vi "g2.vi"() -> ()   [LabVIEW 2020]
uses:
  <vilib>/Math Plots/2D Math Plots/2D Error Bar/2D Error Bar XCtrl/2D Error Bar.xctl
  C:/Program Files/Dotfast Consulting/Timetag Explorer 2.26/ttInterface.dll
  Program Files/Dotfast Consulting/Timetag Explorer 2.26/ttInterface.dll
  <vilib>/Utility/file.llb/Write Delimited Spreadsheet (I64).vi
  <vilib>/Math Plots/2D Math Plots/2D Error Bar/2D Error Bar Datatype/Public/Plot Helper (Fixed).vi
  <vilib>/Math Plots/2D Math Plots/2D Error Bar/2D Error Bar Datatype/2D Error Bar Datatype.lvclass
  <vilib>/Analysis/NI_AALBase.lvlib
panel:
  out "Current Delay":dbl
  out "appended array":i32[](array[numeric])
  out "ABC":refnum<class "2D Plot Datatype.lvclass">[](xcontrol)
  out "Numeric":i32
  in  "Acq Time (s)":dbl=0.1 format="%#_13g"
  out "BC":refnum<class "2D Plot Datatype.lvclass">[](xcontrol)
  in  "# Steps":i32
  in  "stop":bool
  in  "fileName":string
  in  "Folder":path
  in  "CTW in ns":dbl
  out "GetTimeCounter":i32
  out "GetResolution":dbl
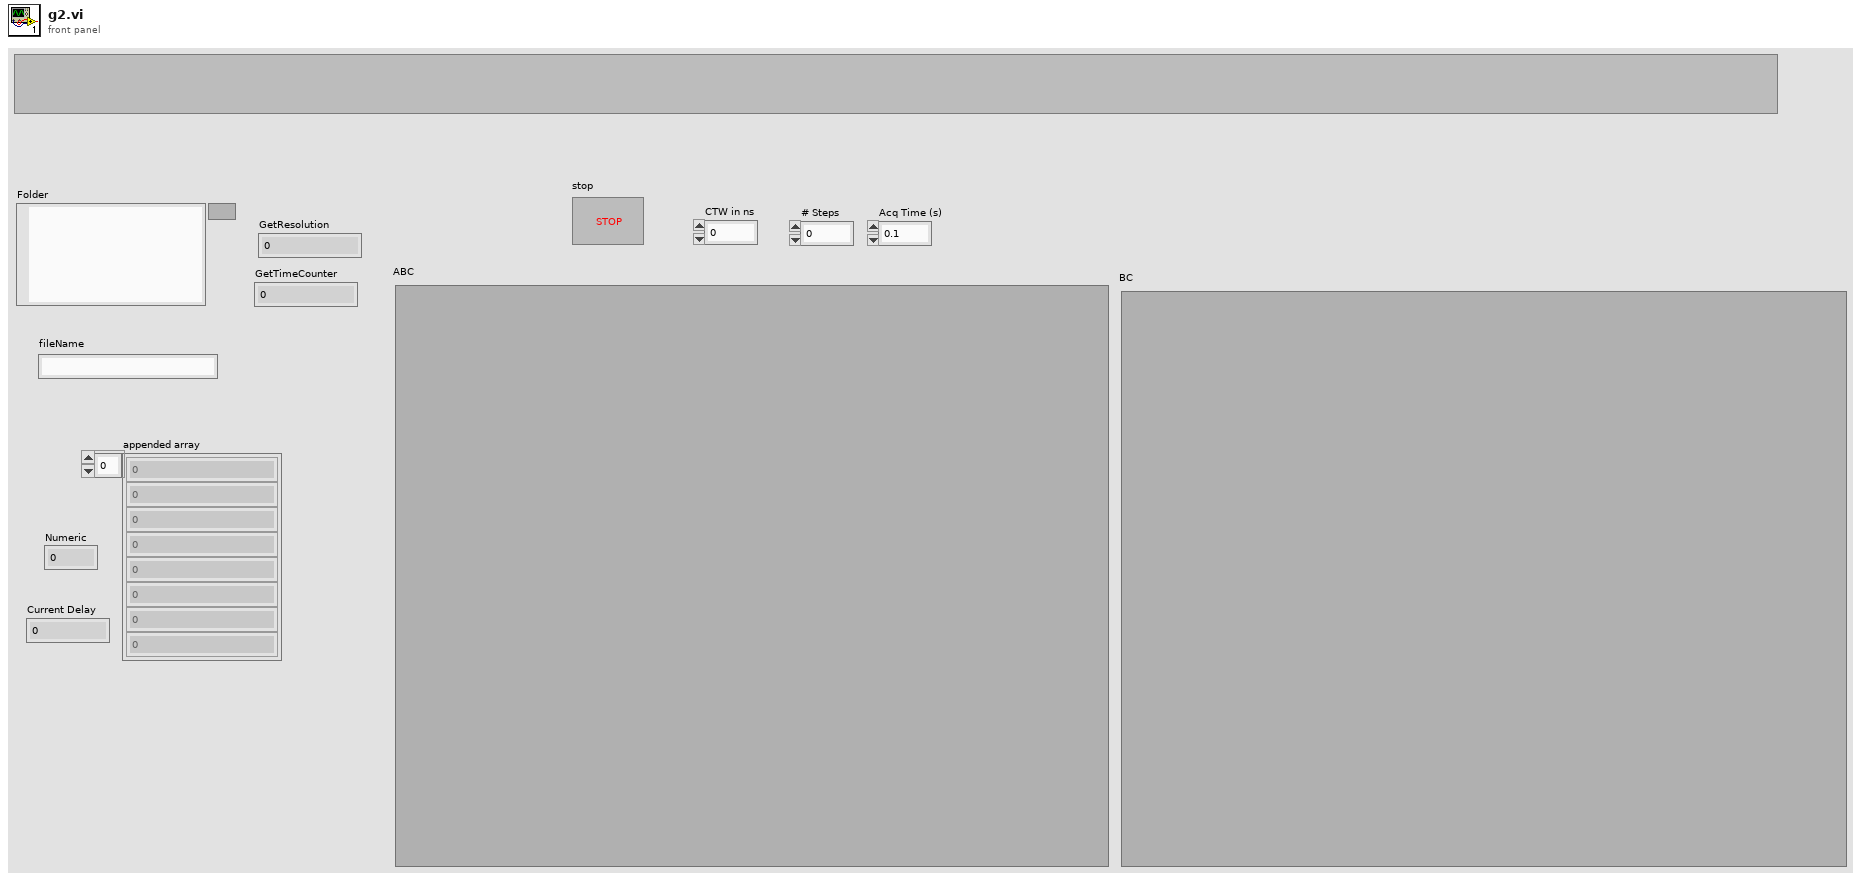
[diagram p1: front panel]
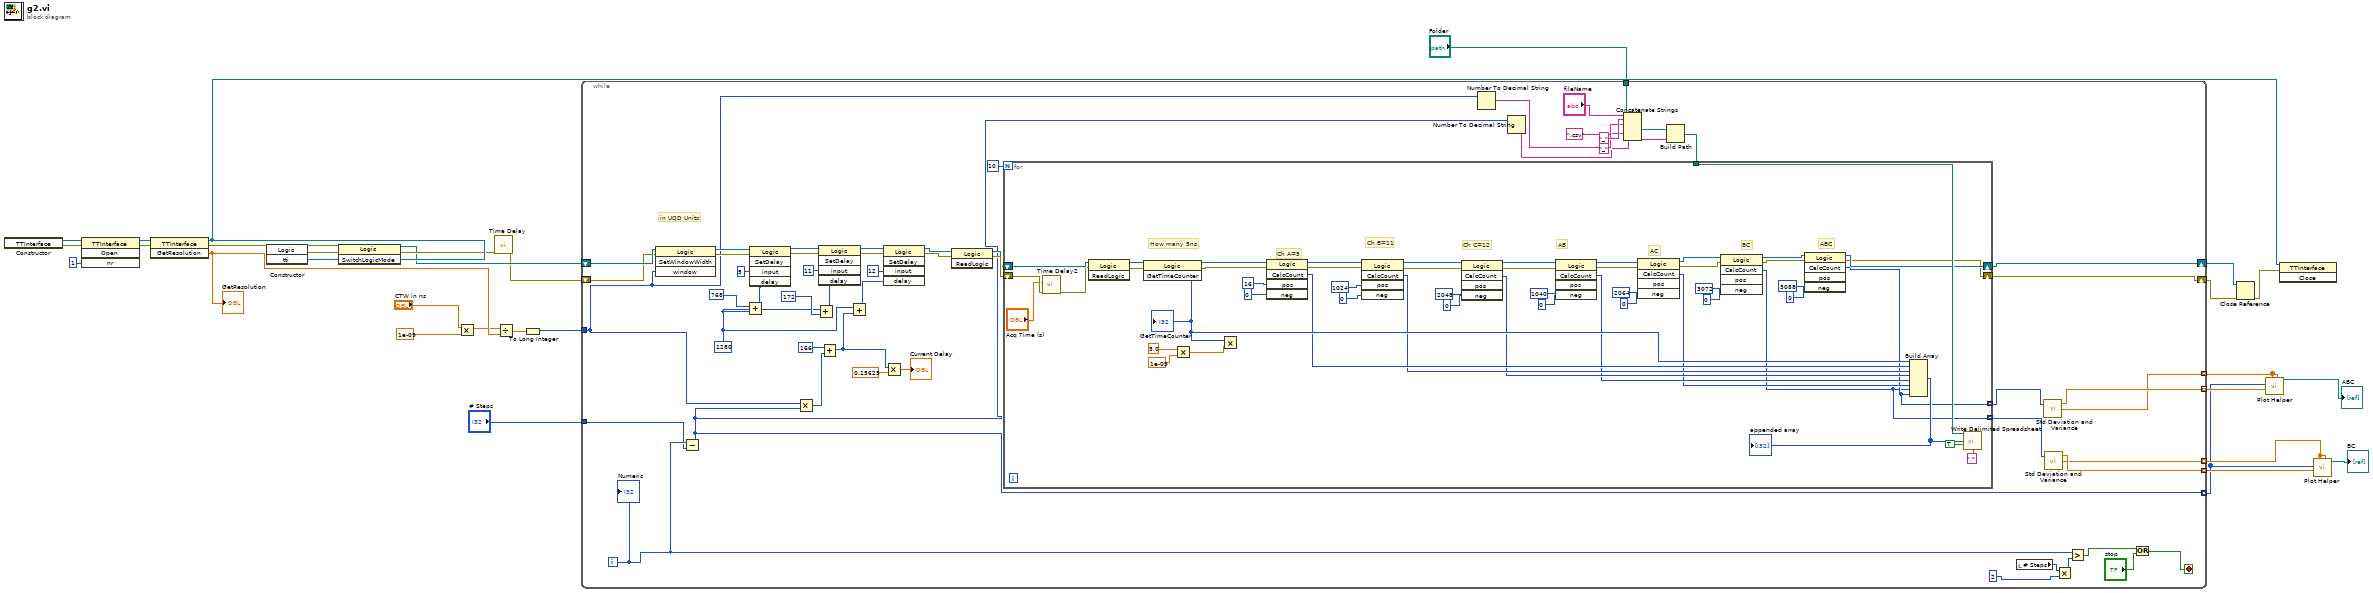
[diagram p0: block diagram]
diagram:
  n1 = constructor class="TTInterface"() -> (reference out=w30:refnum<k24>, error out=w29:errorcluster)  [unwired: 3 in, 1 out]
  n2 = invoke class="TTInterface" method="Open"(reference=w30, error in=w29, "nr"=1) -> (reference out=w26:refnum<k24>, error out=w27:errorcluster)  [unwired: 1 in, 2 out]
  n3 = invoke class="TTInterface" method="GetResolution"(reference=w26, error in=w27) -> (reference out=w25:refnum<k24>, error out=w24:errorcluster, "GetResolution"=w17:dbl)  [unwired: 1 in]
  "GetResolution" <- w17
  n4 = constructor class="Logic"(error in=w24, "tti"=w25) -> (reference out=w23:refnum<k24>, error out=w22:errorcluster)  [unwired: 2 in, 2 out]
  n5 = invoke class="Logic" method="SwitchLogicMode"(reference=w23, error in=w22) -> (reference out=w20:refnum<k24>, error out=w21:errorcluster)  [unwired: 1 in, 1 out]
  n6 = Multiply(x="CTW in ns", y=1e-09) -> (x*y=w16:dbl)
  n7 = call "Time Delay"("error in (no error)"=w21) -> ("error out"=w19:errorcluster)  [unwired: 10 in]
  n8 = Divide(x=w16, y=w17) -> (x/y=w15:dbl)
  n9 = To Long Integer(number=w15) -> (32bit integer=w12:i32)
  n10 = while {
    shift-right: [w54] -> w10
    shift-left: w20 -> [w81]
    shift-right: [w53] -> w9
    shift-left: w19 -> [w80]
    tunnel: "Folder" -> [w75]
    tunnel: w12 -> [w61]
    tunnel: "# Steps" -> [w58]
    tunnel: [w51] -> w7 mode=indexing
    tunnel: [w50] -> w6 mode=indexing
    tunnel: [w49] -> w2 mode=indexing
    tunnel: [w47] -> w4 mode=indexing
    tunnel: [w46] -> w3 mode=indexing
    i -> [w59]
    stop <- w72 stop-if-true
    w31 = 1280
    # "in UQD Units"
    n11 = invoke class="Logic" method="SetWindowWidth"(reference=w81, error in=w80, "window"=w61) -> (reference out=w79:refnum<k24>, error out=w78:errorcluster)  [unwired: 1 in, 2 out]
    n12 = Subtract(x=w59, y=w58) -> (x-y=w49:i32)
    n13 = Add(x=768 ("delay"), y=w31) -> (x+y=w35:i32)
    n14 = invoke class="Logic" method="SetDelay"(reference=w79, error in=w78, "input"=5, "delay"=w35) -> (reference out=w77:refnum<k24>, error out=w76:errorcluster)  [unwired: 1 in, 3 out]
    n15 = Multiply(x=w61, y=w49) -> (x*y=w60:i32)
    n16 = Add(x=w31, y=172 ("delay")) -> (x+y=w33:i32)
    n17 = invoke class="Logic" method="SetDelay"(reference=w77, error in=w76, "input"=11, "delay"=w33) -> (reference out=w69:refnum<k24>, error out=w68:errorcluster)  [unwired: 1 in, 3 out]
    n18 = Add(x=166 ("delay"), y=w60) -> (x+y=w38:i32)
    n19 = Add(x=w31, y=w38) -> (x+y=w32:i32)
    n20 = invoke class="Logic" method="SetDelay"(reference=w69, error in=w68, "input"=12, "delay"=w32) -> (reference out=w67:refnum<k24>, error out=w66:errorcluster)  [unwired: 1 in, 3 out]
    n21 = Multiply(x=w38, y=0.15625) -> (x*y=→"Current Delay":dbl)
    n22 = invoke class="Logic" method="ReadLogic"(reference=w67, error in=w66) -> (reference out=w83:refnum<k24>, error out=w84:errorcluster)  [unwired: 1 in, 1 out]
    n23 = Number To Decimal String(number=w61) -> (decimal integer string=w43:string)  [unwired: 1 in]
    n24 = Number To Decimal String(number=w49) -> (decimal integer string=w41:string)  [unwired: 1 in]
    n25 = Concatenate Strings("fileName", "_" ("string"), w43, "_" ("string"), w41, ".csv" ("string")) -> (w73:string)
    n26 = Build Path(base path=w75, name or relative path=w73) -> (appended path=w74:path)
    n27 = for {
      N: 10 -> [_]
      shift-right: [w94] -> w53
      shift-left: w84 -> [w135]
      shift-right: [w95] -> w54
      shift-left: w83 -> [w134]
      tunnel: w74 -> [w121]
      tunnel: [w86] -> w52 mode=indexing
      tunnel: [w85] -> w48 mode=indexing
      # "ABC"
      # "BC"
      # "AC"
      # "AB"
      # "Ch C=12"
      # "Ch B=11"
      # "Ch A=5"
      # "How many 5ns"
      n28 = call "Time Delay2"("error in (no error)"=w135, "Delay Time (s)"="Acq Time (s)") -> ("error out"=w133:errorcluster)  [unwired: 9 in]
      n29 = invoke class="Logic" method="ReadLogic"(reference=w134, error in=w133) -> (reference out=w128:refnum<k24>, error out=w127:errorcluster)  [unwired: 1 in, 1 out]
      n30 = invoke class="Logic" method="GetTimeCounter"(reference=w128, error in=w127) -> (reference out=w125:refnum<k24>, error out=w124:errorcluster, "GetTimeCounter"=w93:i32)  [unwired: 1 in]
      "GetTimeCounter" <- w93
      n31 = Multiply(x=5.0, y=1e-09) -> (x*y=w129:dbl)
      n32 = Multiply(x=w93, y=w129) -> ()  [unwired: 1 out]
      n33 = invoke class="Logic" method="CalcCount"(reference=w125, error in=w124, "pos"=16, "neg"=0) -> (reference out=w117:refnum<k24>, error out=w116:errorcluster, "CalcCount"=w92:i32)  [unwired: 1 in, 2 out]
      n34 = invoke class="Logic" method="CalcCount"(reference=w117, error in=w116, "pos"=1024, "neg"=0) -> (reference out=w113:refnum<k24>, error out=w112:errorcluster, "CalcCount"=w91:i32)  [unwired: 1 in, 2 out]
      n35 = invoke class="Logic" method="CalcCount"(reference=w113, error in=w112, "pos"=2048, "neg"=0) -> (reference out=w109:refnum<k24>, error out=w108:errorcluster, "CalcCount"=w90:i32)  [unwired: 1 in, 2 out]
      n36 = invoke class="Logic" method="CalcCount"(reference=w109, error in=w108, "pos"=1040, "neg"=0) -> (reference out=w105:refnum<k24>, error out=w104:errorcluster, "CalcCount"=w89:i32)  [unwired: 1 in, 2 out]
      n37 = invoke class="Logic" method="CalcCount"(reference=w105, error in=w104, "pos"=2064, "neg"=0) -> (reference out=w100:refnum<k24>, error out=w101:errorcluster, "CalcCount"=w88:i32)  [unwired: 1 in, 2 out]
      n38 = invoke class="Logic" method="CalcCount"(reference=w100, error in=w101, "pos"=3072, "neg"=0) -> (reference out=w97:refnum<k24>, error out=w96:errorcluster, "CalcCount"=w85:i32)  [unwired: 1 in, 2 out]
      n39 = invoke class="Logic" method="CalcCount"(reference=w97, error in=w96, "pos"=3088, "neg"=0) -> (reference out=w95:refnum<k24>, error out=w94:errorcluster, "CalcCount"=w86:i32)  [unwired: 1 in, 2 out]
      n40 = Build Array(w93, w92, w91, w90, w89, w88, w85, w86) -> (w87:i32[])
      "appended array" <- w87
      n41 = call-poly <vilib>:"Write Delimited Spreadsheet.vi"("file path (dialog if empty)"=w121, "1D data"=w87, "append to file? (new file:F)"=TRUE, "delimiter (\\t)"="," ("delimiter (\\t)")) -> ()  [unwired: 10 in, 2 out]
    }
    n42 = local read "# Steps"() -> (w56:i32)
    n43 = call <vilib>:"Std Deviation and Variance.vi"("X"=w52) -> ("mean"=w51:dbl, "standard deviation"=w50:dbl)  [unwired: 1 in, 1 out]
    n44 = call <vilib>:"Std Deviation and Variance.vi"("X"=w48) -> ("mean"=w47:dbl, "standard deviation"=w46:dbl)  [unwired: 1 in, 1 out]
    n45 = Multiply(x=w56, y=2) -> (x*y=w57:i32)
    n46 = Greater?(x=w59, y=w57) -> (0:w70:bool)
    n47 = Or(x=w70, y="stop") -> (x .or. y?=w72:bool)
    "Numeric" <- w59
  }
  n48 = Close Reference(reference=w10, error in (no error)=w9) -> (error out=w8:errorcluster)
  n49 = call-poly <vilib>:"Plot Helper.vi"("error b vector"=w6, "error a vector"=w6, "y vector"=w7, "x vector"=w2) -> ("2D Plot Class Obj Array out"=→"ABC":refnum<class "2D Plot Datatype.lvclass">[])  [unwired: 2 in, 5 out]
  n50 = invoke class="TTInterface" method="Close"(reference=w25, error in=w8) -> ()  [unwired: 1 in, 3 out]
  n51 = call-poly <vilib>:"Plot Helper.vi"("error b vector"=w3, "error a vector"=w3, "y vector"=w4, "x vector"=w2) -> ("2D Plot Class Obj Array out"=→"BC":refnum<class "2D Plot Datatype.lvclass">[])  [unwired: 2 in, 5 out]
